vi "Set DebugGUIs.vi"(8 "error in (no error)":errorcluster, 10 "DebugGUIs":bool, 11 "Node in":refnum<class "Node.lvclass">) -> (0 "error out":errorcluster, 3 "Node out":refnum<class "Node.lvclass">)   [LabVIEW 2020, in "VolatusConfig.lvlib" / "Node.lvclass"]
uses:
  Node.lvclass
  Node.lvclass/Node.ctl
  VolatusConfigElement/VolatusConfigElement.lvclass
  lv-cdm/CDM-Config/Config Element/Config Element.lvclass
  lv-cdm/CDM-Config/Value Type.ctl
  lv-cdm/CDM-Config/CDM-Config.lvlib
  C:/dev/lv20CE/relink/lv-volatus/VolatusConfig/VolatusConfigElement/VolatusConfigElement.lvclass
  C:/dev/lv20CE/relink/lv-volatus/VolatusConfig/Node/Node.lvclass
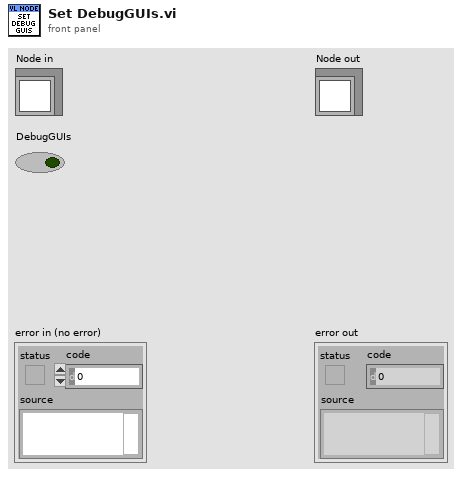
[diagram p1: front panel]
types:
  T1 = typedef "CDM-Config.lvlib/Value Type.ctl" = enum16{"String", "Number", "Bool", "Object", "Array"}
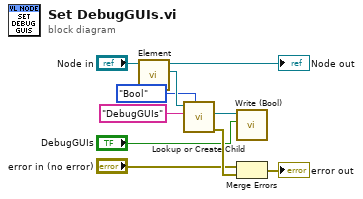
[diagram p0: block diagram]
diagram:
  n1 = call "Element.vi"("VolatusConfigElement in"="Node in") -> ("Element"=w6:refnum<class "Config Element.lvclass">, "VolatusConfigElement out"=→"Node out":refnum<class "Node.lvclass">)  [unwired: 9 in]
  n2 = call "Lookup or Create Child.vi"("Value Type (String)"=Value_Type."Bool", "Name"="DebugGUIs", "Config Element in"=w6) -> ("error out"=w10:errorcluster, "Child"=w3:refnum<class "Config Element.lvclass">)  [unwired: 5 in, 2 out]
  n3 = call "Write (Bool).vi"("Bool Value"="DebugGUIs", "Config Element in"=w3) -> ()  [unwired: 8 in, 2 out]
  n4 = Merge Errors("error in (no error)", w10) -> (→"error out":errorcluster)
